vi "Get State.vi"(8 "error in (no error)":errorcluster, 11 "Instrument Driver in":refnum<class "Instrument Driver.lvclass">) -> (0 "error out":errorcluster, 1 "Data ready":bool, 2 "Armed":bool, 3 "Instrument Driver out":refnum<class "Instrument Driver.lvclass">, 4 "Availiable Samples":u32, 5 "Finished":bool)   [LabVIEW 2019, in "Instrument Driver.lvclass"]
uses:
  Instrument Driver.lvclass
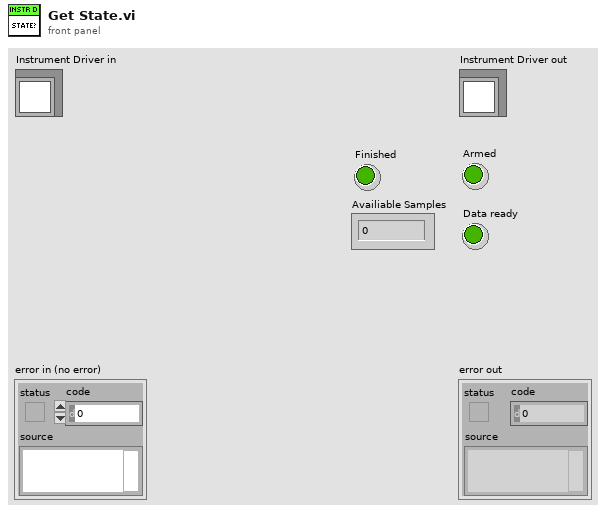
[diagram p1: front panel]
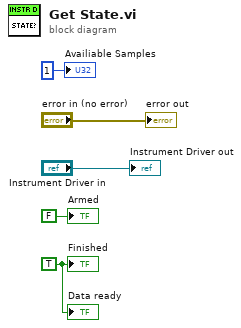
[diagram p0: block diagram]
diagram:
  w3 = TRUE ("Data ready")
  "error out" <- "error in (no error)"
  "Instrument Driver out" <- "Instrument Driver in"
  "Availiable Samples" <- u32 1 ("Availiable Samples")
  "Finished" <- w3
  "Armed" <- FALSE ("Armed")
  "Data ready" <- w3
